vi "WPI_IMU_ADIS16448_ReadRegister.vi"(8 "error in":errorcluster, 10 "Register":u8, 11 "SPIDevRef in":T1={"DevStatus"={"status"=FALSE, "code"=0, "source"=""}, "Handle"=0, "Controller"=enum."Controller 1", "SPI Bus"=enum."Invalid"}) -> (0 "error out":errorcluster, 2 "Register Value":u16, 3 "SPIDevRef out":T1)   [LabVIEW 2014, in "ADIS16448.lvlib"]
uses:
  ADIS16448.lvlib
  <vilib>/Rock Robotics/WPI/SPI/WPI_SPIDevRef.ctl
  <vilib>/Rock Robotics/SystemInterfaces/Typedef/FPGA_TypedefDigitalModule.ctl
  <vilib>/Rock Robotics/SystemInterfaces/spilib/spi_bus.ctl
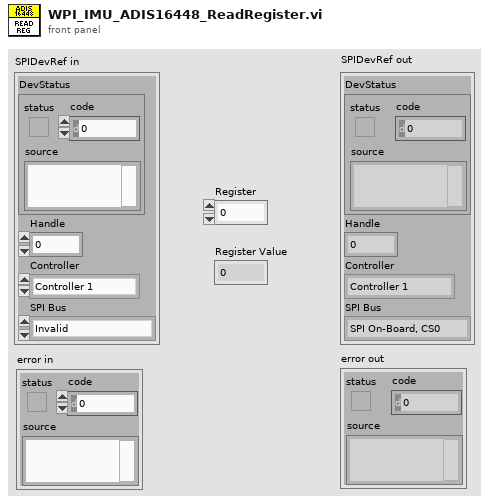
[diagram p1: front panel]
types:
  T1 = typedef "WPI_SPIDevRef.ctl" = cluster{"DevStatus":errorcluster, "Handle":i32, "Controller":T2, "SPI Bus":T3}
  T2 = typedef "FPGA_TypedefDigitalModule.ctl" = enum16{"Controller 1"}
  T3 = typedef "spi_bus.ctl" = enum16{"SPI On-Board, CS0", "SPI On-Board, CS1", "SPI On-Board, CS2", "SPI On-Board, CS3", "SPI MXP", "Invalid"}
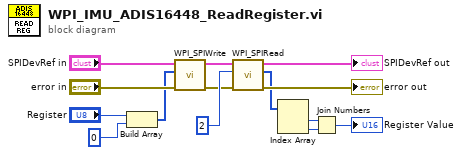
[diagram p0: block diagram]
diagram:
  n1 = Build Array("Register", u8 0 ("element")) -> (w5:u8[])
  n2 = call <vilib>:"WPI_SPIWrite.vi"("error in (no error)"="error in", "Data To Send"=w5, "SPIDevRef"="SPIDevRef in") -> ("error out"=w10:errorcluster, "SPIDevRef"=w13:T1)  [unwired: 6 in, 1 out]
  n3 = call <vilib>:"WPI_SPIRead.vi"("error in (no error)"=w10, "Num to Read"=2, "SPIDevRef"=w13) -> ("error out"=→"error out":errorcluster, "Received Data"=w4:u8[], "SPIDevRef"=→"SPIDevRef out":T1)  [unwired: 6 in]
  n4 = Index Array(array=w4) -> (element #1=w2:u8, element #2=w3:u8)  [unwired: 2 in]
  n5 = Join Numbers(hi=w2, lo=w3) -> ((hi.lo)=→"Register Value":u16)
